vi "Colour to RGB.vi"(7 "Colour":u32) -> (8 "Colours[R,G,B]":u8[](array[numeric]))   [LabVIEW 2012, in "ColourUpStructures.lvlib"]
uses:
  ColourUpStructures.lvlib
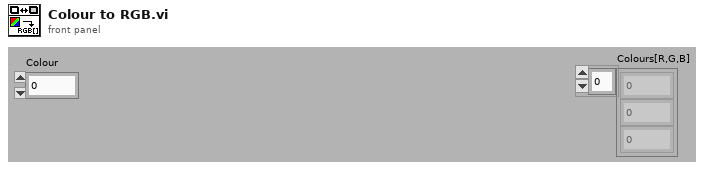
[diagram p1: front panel]
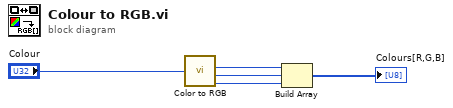
[diagram p0: block diagram]
diagram:
  n1 = call <vilib>:"Color to RGB.vi"("Color"="Colour") -> ("R"=w4:u8, "G"=w3:u8, "B"=w2:u8)  [unwired: 1 out]
  n2 = Build Array(w4, w3, w2) -> (→"Colours[R,G,B]":u8[])
